vi "PrepareRotation.vi"(7 "Rotate amount":dbl=5.0, 8 "error in (no error)":errorcluster, 9 "Acceleration (deg2/s)":dbl=10.0, 10 "Speed (deg/s)":dbl=5.0, 11 "StepperController in":refnum<class "StepperController.lvclass">) -> (0 "error out":errorcluster, 2 "ActualMovement":dbl, 3 "StepperController out":refnum<class "StepperController.lvclass">)   [LabVIEW 2013, in "StepperController.lvclass"]
uses:
  StepperController.lvclass
  StepperController.lvclass/StepperController.ctl
  <vilib>/DAQmx/write.llb/DAQmx Write (Counter 1D Time 1Chan NSamp).vi
  <vilib>/DAQmx/create/channels.llb/DAQmx Create Channel (CO-Pulse Generation-Time).vi
  <vilib>/DAQmx/configure/timing.llb/DAQmx Timing (Implicit).vi
  <vilib>/DAQmx/miscellaneous.llb/DAQmx Fill In Error Info.vi
  <resource>/objmgr/daqmx.rc
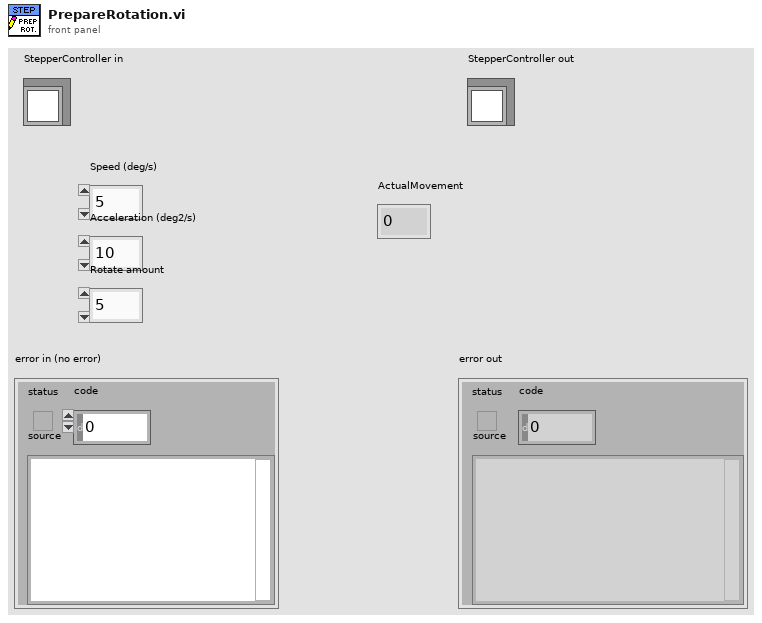
[diagram p1: front panel]
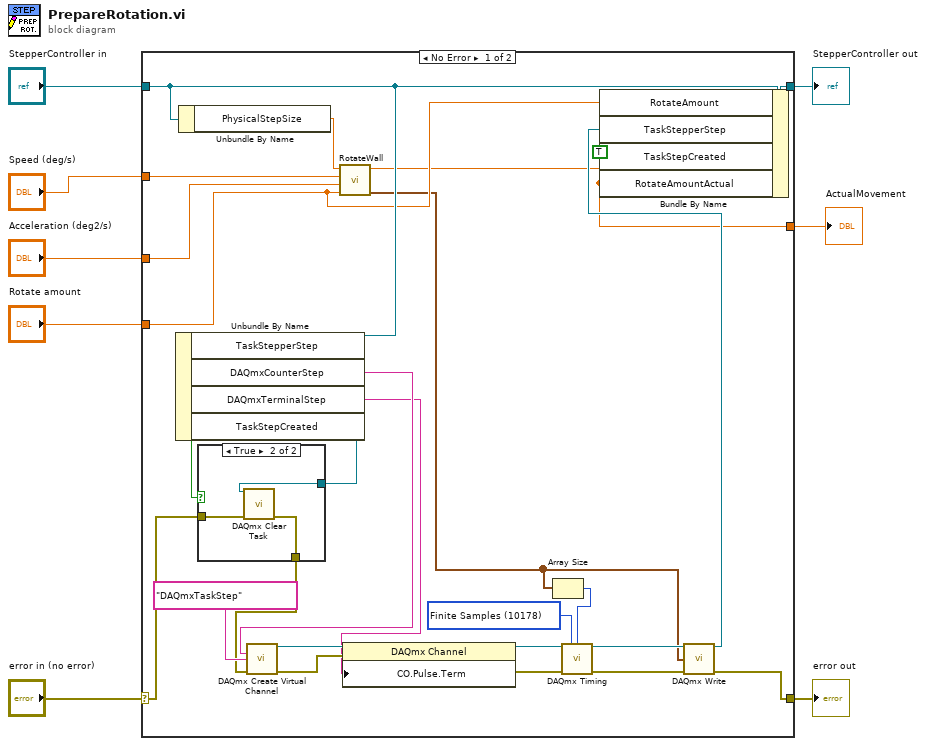
[diagram p0: block diagram]
diagram:
  n1 = case shown="No Error" "error in (no error)" {
    selector: "error in (no error)" -> [w14 w39]
    tunnel: [w21 w39] -> w7
    tunnel: [w19 w40] -> w5
    tunnel: "StepperController in" -> [w20 w40]
    tunnel: "Speed (deg/s)" -> [w33 _]
    tunnel: "Acceleration (deg2/s)" -> [w32 _]
    tunnel: "Rotate amount" -> [w17 _]
    tunnel: [w9 _] -> w1
    frame No Error {
      w25 = 10178 items=["Finite Samples"=10178, "Continuous Samples"=10123, "Hardware Timed Single Point"=12522] ("sample mode")
      n2 = Unbundle By Name(w20) -> ("TaskStepperStep"=w12:refnum<k21>, "DAQmxCounterStep"=w31:tag, "DAQmxTerminalStep"=w28:tag, "TaskStepCreated"=w15:bool)
      n3 = Unbundle By Name(w20) -> ("PhysicalStepSize"=w34:dbl)
      n4 = case shown="True" w15 {
        tunnel: w14 -> [w35 w38]
        tunnel: [w35 w37] -> w13
        tunnel: w12 -> [_ w36]
        frame False {
        }
        frame True {
          n5 = call <vilib>:"DAQmx Clear Task.vi"("task in"=w36, "error in"=w38) -> ("error out"=w37:errorcluster)  [unwired: 13 in]
        }
      }
      n6 = call-poly <vilib>:"DAQmx Create Virtual Channel.vi"("counter"=w31, "name to assign"="DAQmxTaskStep", "error in"=w13) -> ("task out"=w30:refnum<k21>, "error out"=w29:errorcluster)  [unwired: 11 in]
      n7 = call "RotateWall.vi"("Move amount in"=w17, "Acceleration (deg2/s)"=w32, "Speed (deg/s)"=w33, "Physical step size (deg/step)"=w34) -> ("StepTimes"=w11:cluster{dbl, "y":dbl}[], "ActualMovement"=w9:dbl)  [unwired: 6 in]
      n8 = property class="DAQmx Channel"(reference=w30, error in=w29, "CO.Pulse.Term"=w28) -> (reference out=w27:refnum<k21>, error out=w26:errorcluster)
      n9 = Array Size(array=w11) -> (size(s)=w24:i32)
      n10 = call-poly <vilib>:"DAQmx Timing.vi"("task/channels in"=w27, "sample mode"=w25, "samples per channel"=w24, "error in"=w26) -> ("task out"=w23:refnum<k21>, "error out"=w22:errorcluster)  [unwired: 10 in]
      n11 = call-poly <vilib>:"DAQmx Write.vi"("task/channels in"=w23, "data"=w11, "error in"=w22) -> ("task out"=w16:refnum<k21>, "error out"=w21:errorcluster)  [unwired: 10 in, 1 out]
      n12 = Bundle By Name(cluster=w20, "RotateAmount"=w17, "TaskStepperStep"=w16, "TaskStepCreated"=TRUE, "RotateAmountActual"=w9) -> (w19:refnum<class "StepperController.lvclass">)
    }
    frame Error {
    }
  }
  "error out" <- w7
  "StepperController out" <- w5
  "ActualMovement" <- w1
